vi "RemoveFromPlaylist.vi"(8 "error in":errorcluster, 9 "Song Index":i32, 10 "Message Queues":T1, 11 "UI Refs":T2) -> (0 "error out":errorcluster)   [LabVIEW 2015]
uses:
  Controls & Type Defs/UI Data.ctl
  support/Message Queue/All Message Queues.ctl
  support/Message Queue/Message Cluster.ctl
  support/Message Queue/Enqueue Message (Single).vi
  support/Message Queue/Message Queue.lvlib
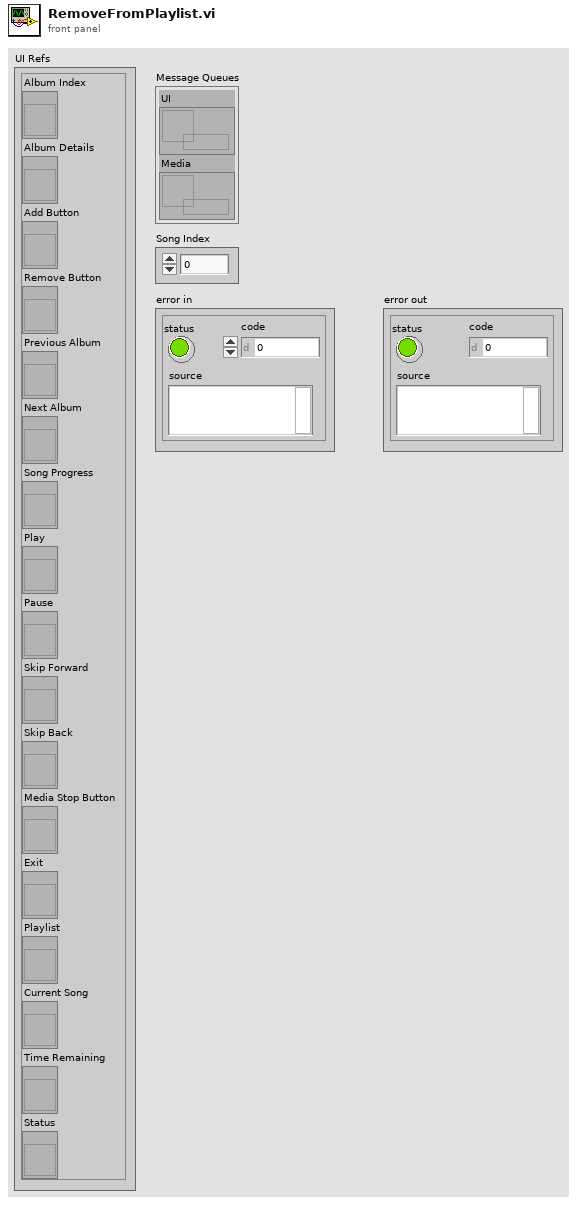
[diagram p1: front panel]
types:
  T1 = typedef "Message Queue.lvlib/All Message Queues.ctl" = cluster{"UI":refnum<queue>, "Media":refnum<queue>}
  T2 = typedef "UI Data.ctl" = cluster{"Album Index":refnum<vi>, "Album Details":refnum<vi>, "Add Button":refnum<vi>, "Remove Button":refnum<vi>, "Previous Album":refnum<vi>, "Next Album":refnum<vi>, "Song Progress":refnum<vi>, "Play":refnum<vi>, "Pause ":refnum<vi>, "Skip Forward":refnum<vi>, "Skip Back":refnum<vi>, "Media Stop Button":refnum<vi>, "Exit":refnum<vi>, "Playlist":refnum<vi>, "Current Song":refnum<vi>, "Time Remaining":refnum<vi>, "Status":refnum<vi>}
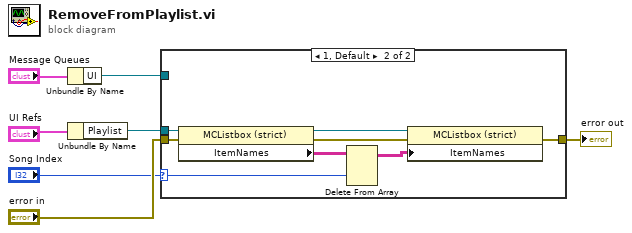
[diagram p0: block diagram]
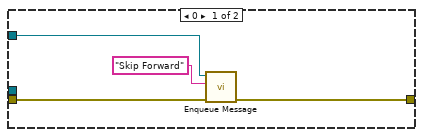
[diagram p2: hidden frame]
diagram:
  n1 = Unbundle By Name("Message Queues") -> ("UI"=w1:refnum<queue>)
  n2 = Unbundle By Name("UI Refs") -> ("Playlist"=w6:refnum<vi>)
  n3 = case shown="1, Default" "Song Index" {
    selector: "Song Index" -> [_ w12]
    tunnel: w6 -> [_ w19]
    tunnel: "error in" -> [w10 w16]
    tunnel: [w9 w14] -> w3
    tunnel: w1 -> [w8 _]
    frame 0 {
      n4 = call-poly "Enqueue Message.vi"("error in (no error)"=w10, "Message"="Skip Forward", "Message Queue"=w8) -> ("error out"=w9:errorcluster)  [unwired: 7 in, 1 out]
    }
    frame 1, Default {
      n5 = property class="MCListbox (strict)"(reference=w19, error in=w16) -> (reference out=w18:refnum<vi>, error out=w17:errorcluster, "ItemNames"=w15:string[][])
      n6 = Delete From Array(array=w15, index (row)=w12) -> (array with subset deleted=w13:string[][])  [unwired: 2 in, 1 out]
      n7 = property class="MCListbox (strict)"(reference=w18, error in=w17, "ItemNames"=w13) -> (error out=w14:errorcluster)  [unwired: 1 out]
    }
  }
  "error out" <- w3
